vi "Min-Max Finder.vi"(3 "Period [s]":sgl=4e-05 format="%#_6p", 4 "Time [sec]":sgl[](array[numeric]) format="%#_6p", 5 "Current/Voltage":sgl[](array[numeric])) -> (0 "Error":bool, 1 "Min Value Per Period":sgl[](array[numeric]), 2 "Max Value Per Period":sgl[](array[numeric]))   [LabVIEW 2016, in "DSI-RT.lvlib"]
uses:
  DSI-RT.lvlib
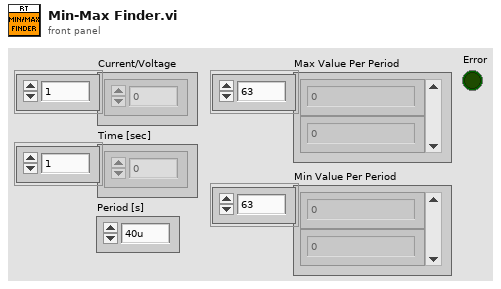
[diagram p1: front panel]
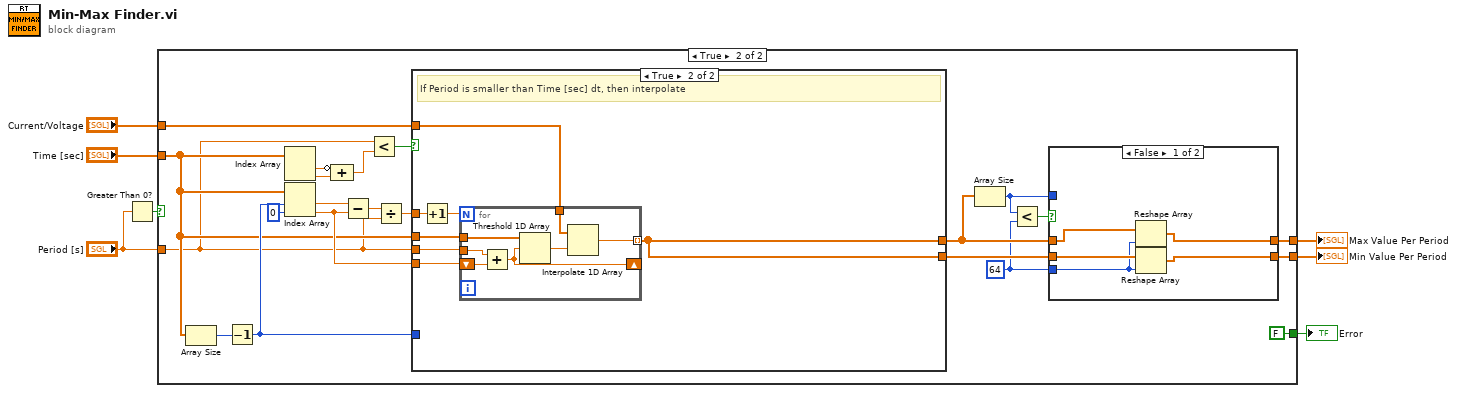
[diagram p0: block diagram]
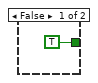
[diagram p2: hidden frame]
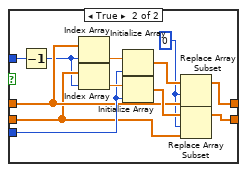
[diagram p3: hidden frame]
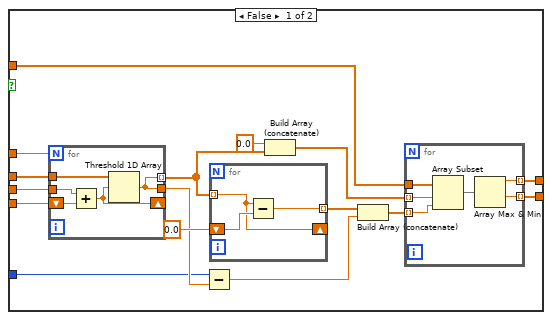
[diagram p4: hidden frame]
diagram:
  n1 = Greater Than 0?(x="Period [s]") -> (x > 0?=w3:bool)
  n2 = case shown="True" w3 {
    tunnel: [_ w11] -> w7
    tunnel: [_ w12] -> w1
    tunnel: "Time [sec]" -> [_ w23]
    tunnel: "Period [s]" -> [_ w19]
    tunnel: "Current/Voltage" -> [_ w17]
    tunnel: [TRUE ("Error") FALSE ("Error")] -> w4
    frame False {
    }
    frame True {
      w10 = 64 ("y")
      n3 = Array Size(array=w23) -> (size(s)=w30:i32)
      n4 = Decrement(x=w30) -> (x-1=w27:i32)
      n5 = Index Array(array=w23) -> (element #1=w21:sgl, element #2=w22:sgl)  [unwired: 2 in]
      n6 = Index Array(array=w23, index #1=w27, index #2=0 ("index")) -> (element #1=w25:sgl, element #2=w24:sgl)
      n7 = Compound Arithmetic op=ADD(invert w21, w22) -> (w20:sgl)
      n8 = Subtract(x=w25, y=w24) -> (x-y=w28:sgl)
      n9 = Less?(x=w19, y=w20) -> (x < y?=w18:bool)
      n10 = Divide(x=w28, y=w19) -> (x/y=w29:sgl)
      n11 = case shown="True" w18 {
        tunnel: w29 -> [w63 w84]
        tunnel: w19 -> [w58 w82]
        tunnel: [w53 w79] -> w14
        tunnel: w23 -> [w52 w83]
        tunnel: [w51 w79] -> w13
        tunnel: w27 -> [w50 _]
        tunnel: w24 -> [w49 w81]
        tunnel: w17 -> [w48 w80]
        frame False {
          n12 = for {
            N: w63 -> [_]
            shift-right: [w75] -> _
            shift-left: w49 -> [w77]
            tunnel: w58 -> [w76]
            tunnel: w52 -> [w74]
            tunnel: [w73] -> w60 mode=indexing
            tunnel: [w73] -> w56
            n13 = Add(x=w76, y=w77) -> (x+y=w75:sgl)
            n14 = Threshold 1D Array(2:w75, 3:w74) -> (0:w73:sgl)  [unwired: 1 in]
          }
          n15 = Subtract(x=w50, y=w56) -> (x-y=w57:sgl)
          n16 = for {
            shift-right: [w71] -> _
            shift-left: sgl 0.0 -> [w72]
            tunnel: w60 -> [w71] mode=indexing
            tunnel: [w70] -> w61 mode=indexing
            n17 = Subtract(x=w71, y=w72) -> (x-y=w70:sgl)
          }
          n18 = Build Array (concatenate)(sgl 0.0, w60) -> (w55:sgl[])
          n19 = Build Array (concatenate)(w61, w57) -> (w54:sgl[])
          n20 = for {
            tunnel: w48 -> [w69]
            tunnel: w55 -> [w68] mode=indexing
            tunnel: w54 -> [w67] mode=indexing
            tunnel: [w65] -> w53 mode=indexing
            tunnel: [w64] -> w51 mode=indexing
            n21 = Array Subset(array=w69, index=w68, length=w67) -> (w66:sgl[])
            n22 = Array Max & Min(array=w66) -> (max value=w65:sgl, min value=w64:sgl)  [unwired: 2 out]
          }
        }
        frame True {
          # "If Period is smaller than Time [sec] dt, then interpolate"
          n23 = Increment(x=w84) -> (x+1=w78:sgl)
          n24 = for {
            N: w78 -> [_]
            shift-right: [w89] -> _
            shift-left: w81 -> [w91]
            tunnel: w82 -> [w90]
            tunnel: w83 -> [w88]
            tunnel: w80 -> [w86]
            tunnel: [w85] -> w79 mode=indexing
            n25 = Add(x=w90, y=w91) -> (x+y=w89:sgl)
            n26 = Threshold 1D Array(2:w89, 3:w88) -> (0:w87:sgl)  [unwired: 1 in]
            n27 = Interpolate 1D Array(1:w87, 2:w86) -> (0:w85:sgl)
          }
        }
      }
      n28 = Array Size(array=w14) -> (size(s)=w9:i32)
      n29 = Less?(x=w9, y=w10) -> (x < y?=w15:bool)
      n30 = case shown="False" w15 {
        tunnel: w14 -> [w35 w39]
        tunnel: w13 -> [w34 w38]
        tunnel: [w33 w42] -> w12
        tunnel: [w32 w43] -> w11
        tunnel: w10 -> [w31 w44]
        tunnel: w9 -> [_ w47]
        frame False {
          n31 = Reshape Array(w35, w31) -> (w32:sgl[])
          n32 = Reshape Array(w34, w31) -> (w33:sgl[])
        }
        frame True {
          w37 = 0 ("index")
          n33 = Decrement(x=w47) -> (x-1=w36:i32)
          n34 = Index Array(array=w39, index=w36) -> (element=w46:sgl)
          n35 = Index Array(array=w38, index=w36) -> (element=w45:sgl)
          n36 = Initialize Array(w46, w44) -> (w41:sgl[])
          n37 = Initialize Array(w45, w44) -> (w40:sgl[])
          n38 = Replace Array Subset(array=w41, new element=w39, index=w37) -> (w43:sgl[])
          n39 = Replace Array Subset(array=w40, new element=w38, index=w37) -> (w42:sgl[])
        }
      }
    }
  }
  "Max Value Per Period" <- w7
  "Min Value Per Period" <- w1
  "Error" <- w4
